vi "Q14070主界面Z100.vi"() -> ()   [LabVIEW 2013]
uses:
  <vilib>/Utility/error.llb/whitespace.ctl
  <vilib>/Utility/file.llb/Write To Spreadsheet File (string).vi
  <vilib>/Utility/file.llb/Write To Spreadsheet File (DBL).vi
  <vilib>/Utility/file.llb/Read From Spreadsheet File (DBL).vi
  <vilib>/Utility/file.llb/Read From Spreadsheet File (string).vi
panel:
  out "放行1":bool
  in  "流水号 3":dbl=22.0 min=1.0 format="%0#8_4g"
  out "打标内容 2":string
  out "PLC":bool
  out "本序已做":bool
  out "10rfid读取完成":bool
  out "10RFID读取触发":bool
  out "FGCS":string
  out "KSJJ":string
  out "10rfid":string
  out "上序不合格":bool
  out "上序合格":bool
  out "自动工步号Z110":dbl
  out "Z110工位操作状态":string
  out "芯片ID":string
  out "本序不合格":bool
  out "权限":string
  out "本序合格":bool
  in  "停止":bool
  in  "自动工步号":dbl
  out "产品选型":dbl
  out "Z100工位操作状态":string
  in  "联线按钮":bool
  in  "选项卡控件":enum32{"自动界面", "手动界面"}(tab)
  out "字符串":string
  in  "批次":string="A"
  in  "流水号 2":dbl=22.0 min=1.0 format="%0#8_4g"
  out "打标内容":string
  out "打标内容第二行":string
  in  "流水号":dbl min=1.0 format="%0#6_4g"
  out "打标内容第一行":string
  in  "放行":bool
  in  "阻挡":bool
  in  "Z110旋转气缸回原":bool
  in  "Z110旋转气缸旋转":bool
  in  "Z100上阻挡器":bool
  in  "Z100下阻挡器":bool
  in  "Z100顶升气缸上升":bool
  in  "Z100顶升气缸下降":bool
  in  "Z110下阻挡器":bool
  in  "Z110顶升气缸上升":bool
  in  "Z110顶升气缸下降":bool
  out "放行按钮":bool
  out "启动按钮":bool
  out "复位按钮":bool
  out "自动手动旋钮":bool
  out "急停按钮":bool
  out "本工位检测":bool
  out "Z110下工位检测":bool
  out "Z110放行按钮":bool
  out "顶升气缸上位":bool
  out "上工位检测":bool
  out "Z110本工位检测":bool
  out "顶升气缸下位":bool
  out "Z110复位按钮":bool
  out "Z110旋转原位":bool
  out "Z110急停按钮":bool
  out "下工位检测":bool
  out "Z110顶升下位":bool
  out "Z110顶升上位":bool
  out "Z110旋转位":bool
  in  "打标完成":bool
  out "员工ID":string
  out "员工姓名":string
  in  "型号选择":u16(ring)=1 items=["J709", "J706", "J728"]
  in  "参数加载":bool
  out "产品ID":string="4BSHL07134CCA"
  # "芜湖机械转向器装配线"
  # "激光打标"
  # "Q14070机械转向器装配线"
  # "湖北唯思凌科装备制造有限公司 设计开发 (C)2015"
  # "J728"
  # "J709"
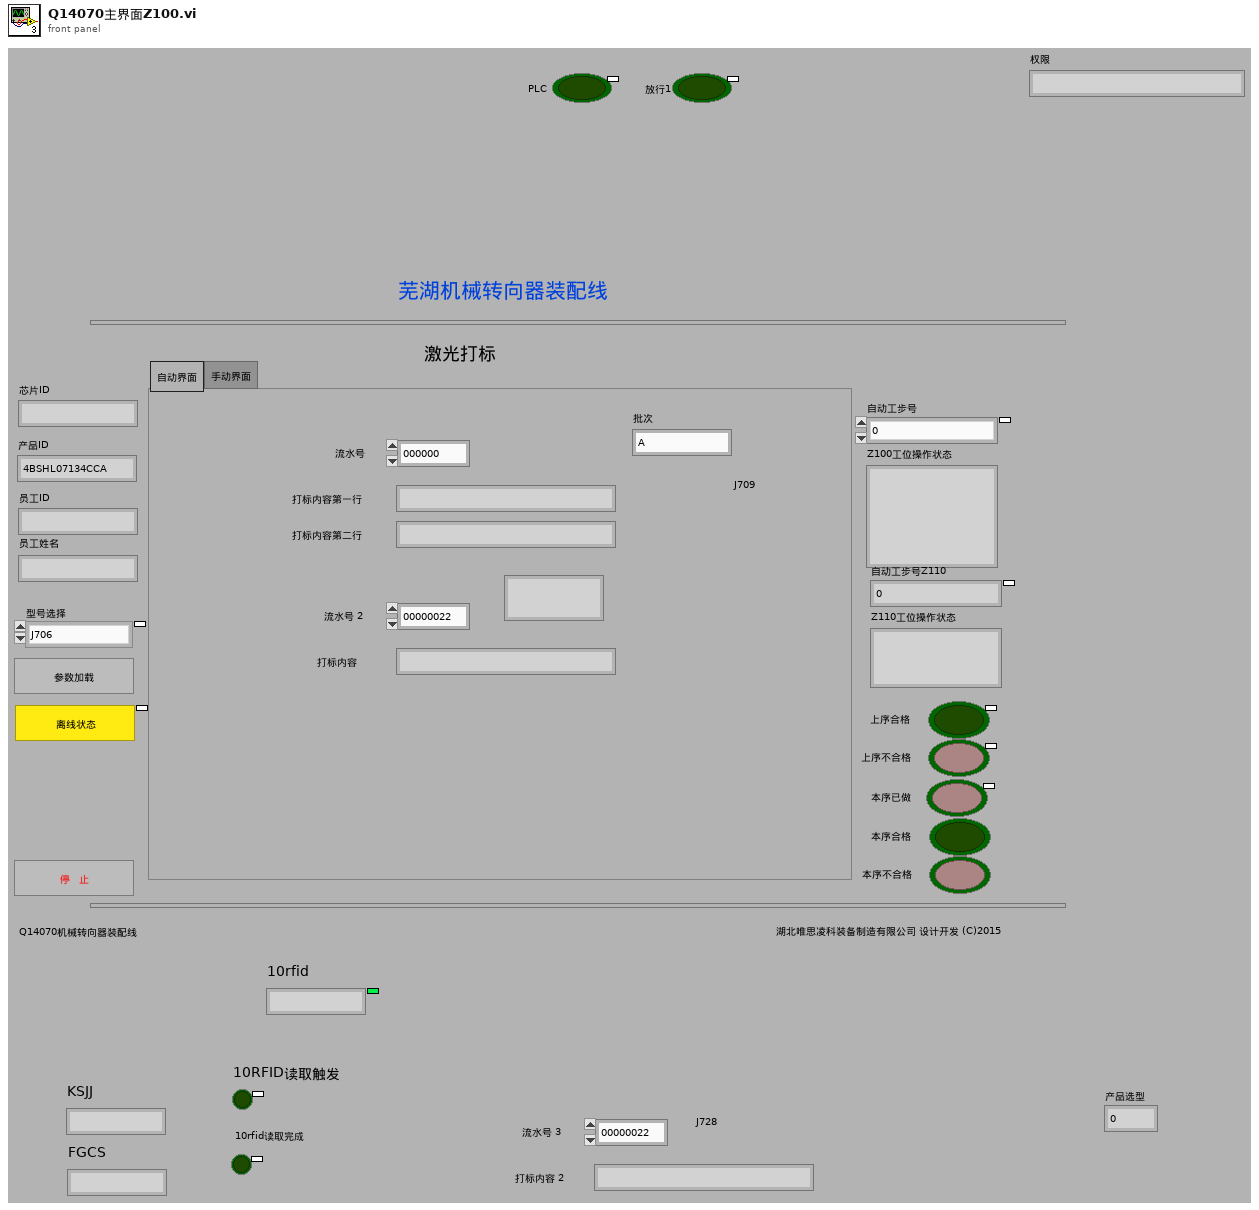
[diagram p1: front panel]
types:
  T1 = enum16{"open", "replace", "create", "open or create", "replace or create", "replace or create with confirmation"}
  T2 = typedef "whitespace.ctl" = u16
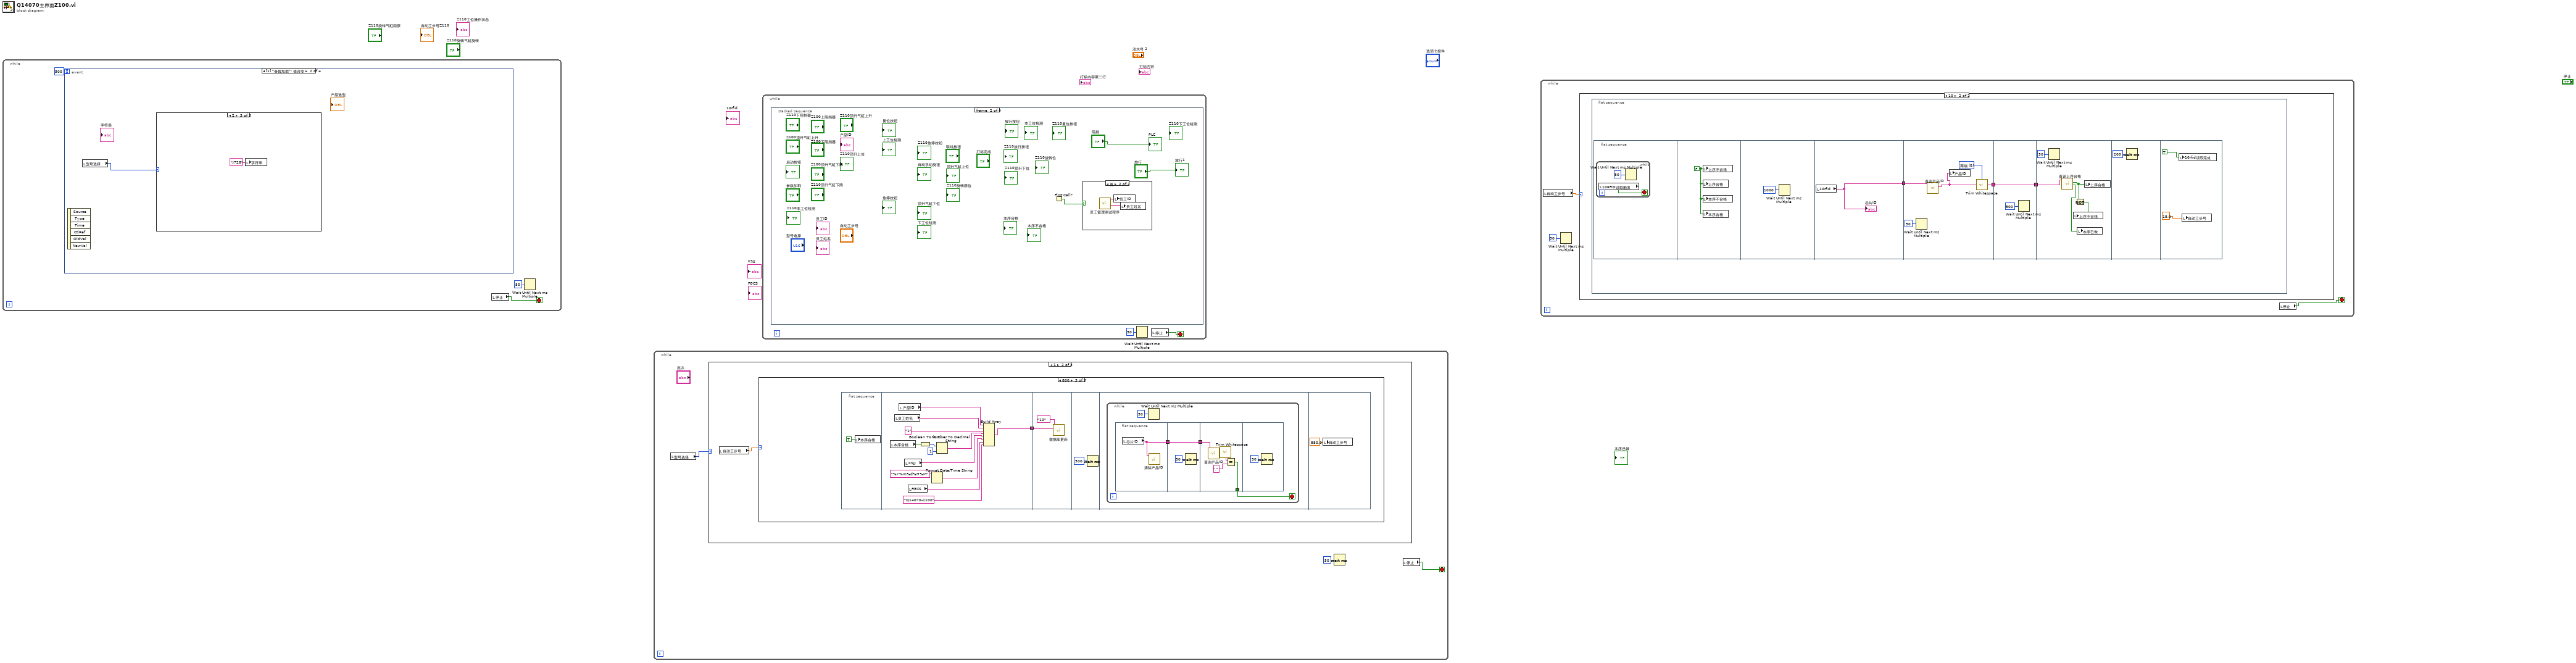
[diagram p0: block diagram]
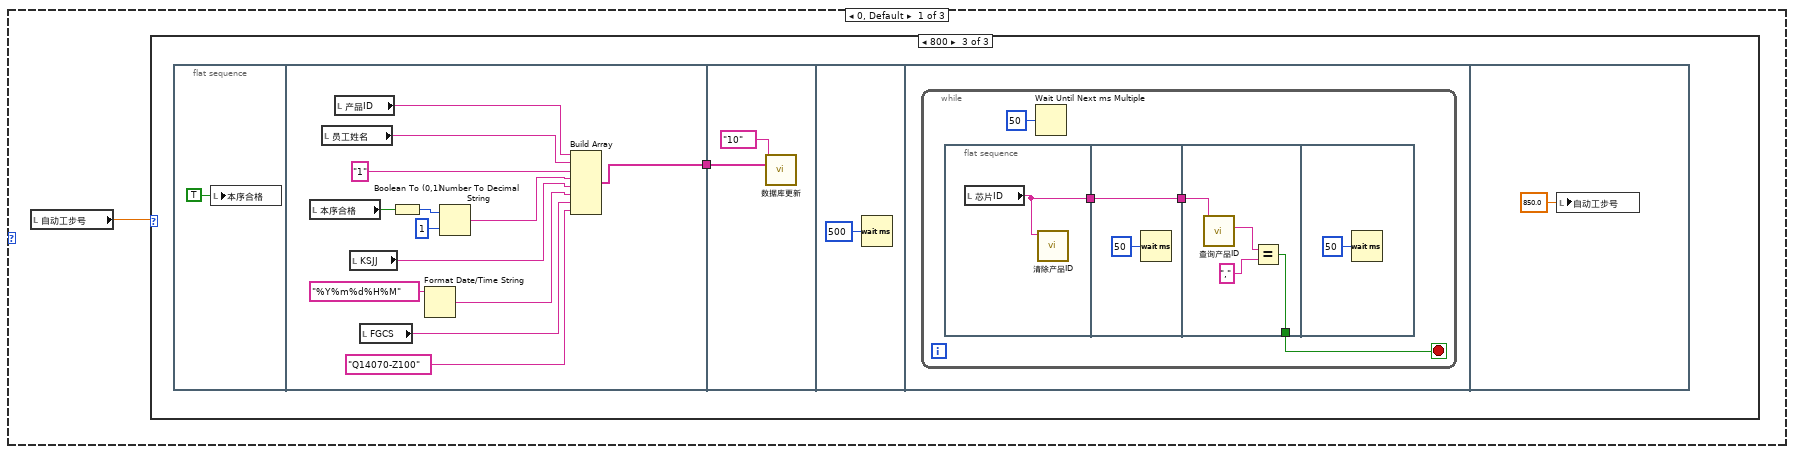
[diagram p2: hidden frame]
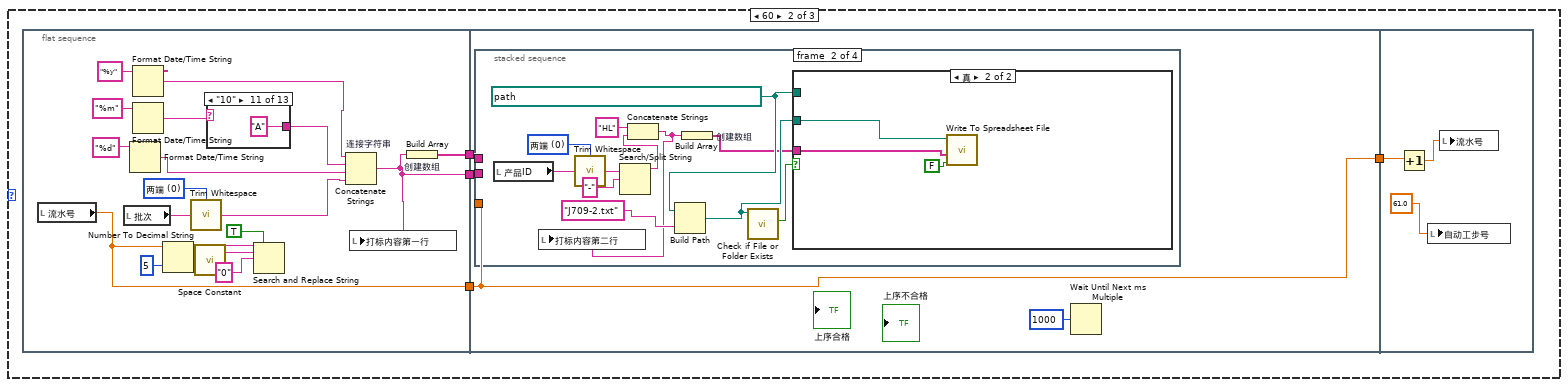
[diagram p4: hidden frame]
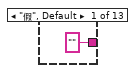
[diagram p5: hidden frame]
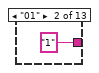
[diagram p6: hidden frame]
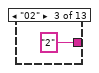
[diagram p7: hidden frame]
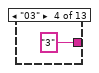
[diagram p8: hidden frame]
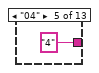
[diagram p9: hidden frame]
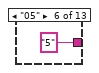
[diagram p10: hidden frame]
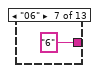
[diagram p11: hidden frame]
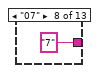
[diagram p12: hidden frame]
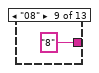
[diagram p13: hidden frame]
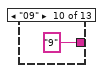
[diagram p14: hidden frame]
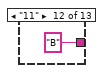
[diagram p15: hidden frame]
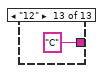
[diagram p16: hidden frame]
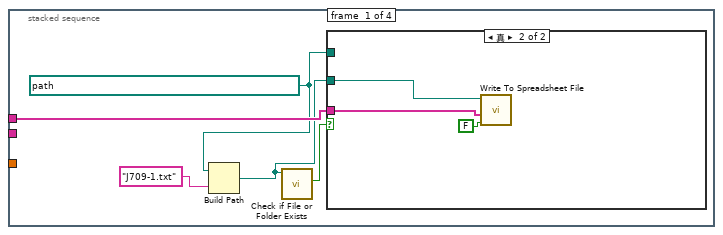
[diagram p17: hidden frame]
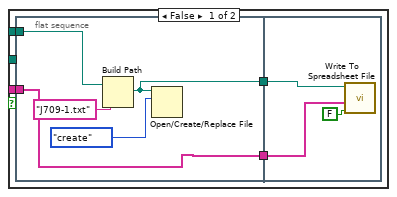
[diagram p18: hidden frame]
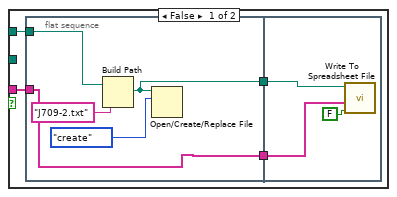
[diagram p19: hidden frame]
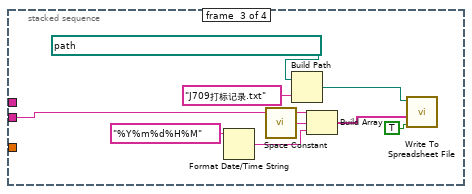
[diagram p20: hidden frame]
diagram:
  n1 = while {
    stop <- w1 stop-if-true
    n2 = event shown="[1] \"参数加载\": 值改变" {
      selector: _ -> [_ _ _ _]
      dyn-events: _ -> [_ _ _ _]
      timeout: 500 -> [_ _ _ _]
      event Timeout {
        n3 = event-data() -> ()  [unwired: 3 out]
      }
      event "参数加载": Value Change {
        n4 = event-data() -> ()  [unwired: 7 out]
        n5 = local read "型号选择"() -> (w4:u16)
        n6 = case shown="2" w4 {
          frame 0, Default {
          }
          frame 1 {
            n7 = local write "字符串"("J706" ("字符串")) -> ()
          }
          frame 2 {
            n8 = local write "字符串"("J728" ("字符串")) -> ()
          }
        }
      }
      event "停止": Value Change {
        n9 = event-data() -> ()  [unwired: 7 out]
        n10 = flat-sequence {
          frame #0 {
          }
          frame #1 {
            n11 = Wait Until Next ms Multiple(millisecond multiple=u32 1000 ("毫秒倍数")) -> ()  [unwired: 1 out]
          }
          frame #2 {
            n12 = Quit LabVIEW(quit? (T)=TRUE ("停止？(T)")) -> ()
          }
        }
      }
      event "产品ID": Value Change {
        n13 = event-data() -> ()  [unwired: 7 out]
        n14 = Format Date/Time String(time format string (%c)="%Y%m%d%H%M" ("时间格式字符串(%c)")) -> (date/time string=w9:string)  [unwired: 2 in]
        n15 = local write "KSJJ"(w9) -> ()
      }
    }
    n16 = local read "停止"() -> (w1:bool)
    n17 = Wait Until Next ms Multiple(millisecond multiple=u32 50 ("毫秒倍数")) -> ()  [unwired: 1 out]
  }
  n18 = while {
    stop <- w12 stop-if-true
    n19 = local read "型号选择"() -> (w13:u16)
    n20 = case shown="1" w13 {
      frame 0, Default {
        n21 = local read "自动工步号"() -> (w14:dbl)
        n22 = case shown="800" w14 {
          frame 0, Default {
          }
          frame 60 {
            n23 = flat-sequence {
              tunnel: [w31] -> w18
              tunnel: [w30] -> w17
              tunnel: [w20] -> w15
              tunnel: [w51] -> w16
              tunnel: w18 -> [w52]
              tunnel: w17 -> [w51]
              tunnel: w15 -> [w50]
              tunnel: w16 -> [w119]
              frame #0 {
                w25 = T2 0 items=["两端", "字符串首端", "字符串末端"] ("location (both)")
                n24 = local read "流水号"() -> (w30:dbl)
                n25 = local read "批次"() -> (w26:string)
                n26 = Format Date/Time String(time format string (%c)="%d" ("时间格式字符串(%c)")) -> (date/time string=w22:string)  [unwired: 2 in]
                n27 = Format Date/Time String(time format string (%c)="%y" ("时间格式字符串(%c)")) -> (date/time string=w19:string)  [unwired: 2 in]
                n28 = Format Date/Time String(time format string (%c)="%m" ("时间格式字符串(%c)")) -> (date/time string=w27:string)  [unwired: 2 in]
                n29 = Number To Decimal String(number=w30, width (-)=i16 5 ("宽度(-)")) -> (decimal integer string=w33:string)
                n30 = call <vilib>:"Trim Whitespace.vi"("string"=w26, "location (both)"=w25) -> ("trimmed string"=w21:string)
                n31 = call <vilib>:"Space Constant.vi"() -> ("String"=w35:string)
                n32 = case shown="\"10\"" w27 {
                  tunnel: ["" "1" "2" "3" "4" "5" "6" "7" "8" "9" "A" "B" "C"] -> w23
                  frame "假", Default {
                  }
                  frame "01" {
                  }
                  frame "02" {
                  }
                  frame "03" {
                  }
                  frame "04" {
                  }
                  frame "05" {
                  }
                  frame "06" {
                  }
                  frame "07" {
                  }
                  frame "08" {
                  }
                  frame "09" {
                  }
                  frame "10" {
                  }
                  frame "11" {
                  }
                  frame "12" {
                  }
                }
                n33 = Search and Replace String(replace all?=TRUE ("替换全部？(F)"), input string=w33, search string=w35, replace string="0" ("替换字符串(\"\")")) -> ()  [unwired: 4 in, 4 out]
                n34 = Concatenate Strings "连接字符串"(w19, w23, w22, w21) -> (w20:string)
                n35 = local write "打标内容第一行"(w20) -> ()
                n36 = Build Array "创建数组"(w20) -> (w31:string[])
              }
              frame #1 {
                n37 = stacked-sequence {
                  tunnel: w52 -> [w57 _ _ _]
                  tunnel: w51 -> [_ _ _ w112]
                  tunnel: w50 -> [_ _ w101 _]
                  frame #0 {
                    w55 = path "D:/Q14070-Z100人机界面/子VI/打标内容/J709" ("file path (dialog if empty)")
                    n38 = Build Path(base path=w55, name or relative path="J709-1.txt" ("名称或相对路径")) -> (appended path=w56:path)
                    n39 = call <vilib>:"Check if File or Folder Exists.vi"("path"=w56) -> ("file or folder exists?"=w58:bool)  [unwired: 8 in, 2 out]
                    n40 = case shown="真" w58 {
                      tunnel: w56 -> [_ w73]
                      tunnel: w55 -> [w62 _]
                      tunnel: w57 -> [w59 w71]
                      frame False {
                        n41 = flat-sequence {
                          tunnel: w62 -> [w67]
                          tunnel: [w64] -> w61
                          tunnel: [w63] -> w60
                          tunnel: w59 -> [w63]
                          tunnel: w61 -> [w69]
                          tunnel: w60 -> [w68]
                          frame #0 {
                            n42 = Build Path(base path=w67, name or relative path="J709-1.txt" ("名称或相对路径")) -> (appended path=w64:path)
                            n43 = Open/Create/Replace File ("打开/创建/替换文件")(file path (use dialog)=w64, operation (0:open)=T1."create" ("操作(0:open)")) -> ()  [unwired: 4 in, 3 out]
                          }
                          frame #1 {
                            n44 = call-poly <vilib>:"Write To Spreadsheet File.vi"("append to file? (new file:F)"=FALSE, "1D data"=w68, "file path (dialog if empty)"=w69) -> ()  [unwired: 5 in, 1 out]
                          }
                        }
                      }
                      frame True {
                        n45 = call-poly <vilib>:"Write To Spreadsheet File.vi"("append to file? (new file:F)"=FALSE, "1D data"=w71, "file path (dialog if empty)"=w73) -> ()  [unwired: 5 in, 1 out]
                      }
                    }
                  }
                  frame #1 {
                    w81 = T2 0 items=["两端", "字符串首端", "字符串末端"] ("location (both)")
                    w83 = path "D:/Q14070-Z100人机界面/子VI/打标内容/J709" ("file path (dialog if empty)")
                    n46 = local read "产品ID"() -> (w80:string)
                    n47 = call <vilib>:"Trim Whitespace.vi"("string"=w80, "location (both)"=w81) -> ("trimmed string"=w76:string)
                    n48 = Search/Split String(string=w76, search string/char (-)="-" ("搜索字符串/字符(-)")) -> (substring before match=w75:string)  [unwired: 1 in, 2 out]
                    n49 = Concatenate Strings ("连接字符串")("HL" ("字符串"), w75) -> (w77:string)
                    n50 = local write "打标内容第二行"(w77) -> ()
                    n51 = Build Path(base path=w83, name or relative path="J709-2.txt" ("名称或相对路径")) -> (appended path=w84:path)
                    n52 = Build Array "创建数组"(w77) -> (w78:string[])
                    n53 = call <vilib>:"Check if File or Folder Exists.vi"("path"=w84) -> ("file or folder exists?"=w85:bool)  [unwired: 8 in, 2 out]
                    n54 = case shown="真" w85 {
                      tunnel: w84 -> [_ w100]
                      tunnel: w83 -> [w89 _]
                      tunnel: w78 -> [w86 w98]
                      frame False {
                        n55 = flat-sequence {
                          tunnel: w89 -> [w94]
                          tunnel: [w92] -> w88
                          tunnel: [w91] -> w87
                          tunnel: w86 -> [w91]
                          tunnel: w88 -> [w96]
                          tunnel: w87 -> [w95]
                          frame #0 {
                            n56 = Build Path(base path=w94, name or relative path="J709-2.txt" ("名称或相对路径")) -> (appended path=w92:path)
                            n57 = Open/Create/Replace File ("打开/创建/替换文件")(file path (use dialog)=w92, operation (0:open)=T1."create" ("操作(0:open)")) -> ()  [unwired: 4 in, 3 out]
                          }
                          frame #1 {
                            n58 = call-poly <vilib>:"Write To Spreadsheet File.vi"("append to file? (new file:F)"=FALSE, "1D data"=w95, "file path (dialog if empty)"=w96) -> ()  [unwired: 5 in, 1 out]
                          }
                        }
                      }
                      frame True {
                        n59 = call-poly <vilib>:"Write To Spreadsheet File.vi"("append to file? (new file:F)"=FALSE, "1D data"=w98, "file path (dialog if empty)"=w100) -> ()  [unwired: 5 in, 1 out]
                      }
                    }
                  }
                  frame #2 {
                    n60 = Format Date/Time String(time format string (%c)="%Y%m%d%H%M" ("时间格式字符串(%c)")) -> (date/time string=w104:string)  [unwired: 2 in]
                    n61 = call <vilib>:"Space Constant.vi"() -> ("String"=w105:string)
                    n62 = Build Path(base path=path "D:/Q14070-Z100人机界面/子VI/打标内容/J709" ("file path (dialog if empty)"), name or relative path="J709打标记录.txt" ("名称或相对路径")) -> (appended path=w102:path)
                    n63 = Build Array(w101, w105, w104) -> (w103:string[])
                    n64 = call-poly <vilib>:"Write To Spreadsheet File.vi"("append to file? (new file:F)"=TRUE, "1D data"=w103, "file path (dialog if empty)"=w102) -> ()  [unwired: 5 in, 1 out]
                  }
                  frame #3 {
                    n65 = Increment(x=w112) -> (x+1=w111:dbl)
                    n66 = Build Array(w111) -> (w110:dbl[])
                    n67 = Build Path(base path=path "D:/Q14070-Z100人机界面/子VI/打标内容/J709" ("file path (dialog if empty)"), name or relative path="J709流水号.txt" ("名称或相对路径")) -> (appended path=w113:path)
                    n68 = call-poly <vilib>:"Write To Spreadsheet File.vi"("append to file? (new file:F)"=FALSE, "1D data"=w110, "file path (dialog if empty)"=w113) -> ()  [unwired: 5 in, 1 out]
                  }
                }
                n69 = Wait Until Next ms Multiple(millisecond multiple=u32 1000 ("毫秒倍数")) -> ()  [unwired: 1 out]
              }
              frame #2 {
                n70 = Increment(x=w119) -> (x+1=w118:dbl)
                n71 = local write "自动工步号"(61.0 ("打标工位工步号")) -> ()
                n72 = local write "流水号"(w118) -> ()
              }
            }
          }
          frame 800 {
            n73 = flat-sequence {
              tunnel: [w123] -> w120
              tunnel: w120 -> [w135]
              frame #0 {
                n74 = local write "本序合格"(TRUE ("本序合格")) -> ()
              }
              frame #1 {
                n75 = local read "本序合格"() -> (w122:bool)
                n76 = local read "员工姓名"() -> (w130:string)
                n77 = local read "产品ID"() -> (w131:string)
                n78 = local read "KSJJ"() -> (w127:string)
                n79 = local read "FGCS"() -> (w125:string)
                n80 = Boolean To (0,1)(Boolean=w122) -> (0, 1=w134:i16)
                n81 = Format Date/Time String(time format string (%c)="%Y%m%d%H%M" ("时间格式字符串(%c)")) -> (date/time string=w126:string)  [unwired: 2 in]
                n82 = Number To Decimal String(number=w134, width (-)=i16 1 ("宽度(-)")) -> (decimal integer string=w128:string)
                n83 = Build Array(w131, w130, "1", w128, w127, w126, w125, "Q14070-Z100") -> (w123:string[])
              }
              frame #2 {
                n84 = call "数据库更新.vi"("设备号"="10", "数据"=w135) -> ()  [unwired: 13 in, 1 out]
              }
              frame #3 {
                n85 = Wait (ms)(milliseconds to wait=u32 500 ("等待时间（毫秒）")) -> ()  [unwired: 1 out]
              }
              frame #4 {
                n86 = while {
                  stop <- w138 stop-if-true
                  n87 = flat-sequence {
                    tunnel: [w142] -> w139
                    tunnel: [w143] -> w140
                    tunnel: w139 -> [w143]
                    tunnel: w140 -> [w148]
                    tunnel: [w145] -> w138
                    frame #0 {
                      n88 = local read "芯片ID"() -> (w142:string)
                      n89 = call "清除产品ID.vi"("芯片编码"=w142) -> ()  [unwired: 10 in, 1 out]
                    }
                    frame #1 {
                      n90 = Wait (ms)(milliseconds to wait=u32 50 ("等待时间（毫秒）")) -> ()  [unwired: 1 out]
                    }
                    frame #2 {
                      n91 = call "查询产品ID.vi"("芯片编码"=w148) -> ("产品ID"=w146:string)  [unwired: 8 in, 2 out]
                      n92 = Equal?(x=w146, y=",") -> (x = y?=w145:bool)
                    }
                    frame #3 {
                      n93 = Wait (ms)(milliseconds to wait=u32 50 ("等待时间（毫秒）")) -> ()  [unwired: 1 out]
                    }
                  }
                  n94 = Wait Until Next ms Multiple(millisecond multiple=u32 50 ("毫秒倍数")) -> ()  [unwired: 1 out]
                }
              }
              frame #5 {
                n95 = local write "自动工步号"(850.0 ("自动工步号")) -> ()
              }
            }
          }
        }
      }
      frame 1 {
        n96 = local read "自动工步号"() -> (w151:dbl)
        n97 = case shown="800" w151 {
          frame 0, Default {
          }
          frame 60 {
            n98 = flat-sequence {
              tunnel: [w164] -> w156
              tunnel: [w163] -> w155
              tunnel: [w162] -> w154
              tunnel: [w171] -> w153
              tunnel: w156 -> [w173]
              tunnel: w155 -> [w171]
              tunnel: w154 -> [w172]
              tunnel: w153 -> [w212]
              tunnel: [w212] -> w152
              tunnel: w152 -> [w215]
              frame #0 {
                w160 = T2 0 items=["两端", "字符串首端", "字符串末端"] ("location (both)")
                n99 = local read "产品ID"() -> (w161:string)
                n100 = local read "流水号 2"() -> (w163:dbl)
                n101 = call <vilib>:"Trim Whitespace.vi"("string"=w161, "location (both)"=w160) -> ("trimmed string"=w159:string)
                n102 = Format Date/Time String(time format string (%c)="%y%m" ("时间格式字符串(%c)")) -> ()  [unwired: 2 in, 1 out]
                n103 = Number To Decimal String(number=w163, width (-)=i16 5 ("宽度(-)")) -> (decimal integer string=w166:string)
                n104 = call <vilib>:"Space Constant.vi"() -> ("String"=w168:string)
                n105 = Search/Split String(string=w159, search string/char (-)="-" ("搜索字符串/字符(-)")) -> (substring before match=w157:string)  [unwired: 1 in, 2 out]
                n106 = Search and Replace String(replace all?=TRUE ("替换全部？(F)"), input string=w166, search string=w168, replace string="0" ("替换字符串(\"\")")) -> ()  [unwired: 4 in, 4 out]
                n107 = Concatenate Strings "连接字符串"(w157) -> (w162:string)
                n108 = local write "打标内容"(w162) -> ()
                n109 = Build Array(w162) -> (w164:string[])
              }
              frame #1 {
                n110 = stacked-sequence {
                  tunnel: w173 -> [w178 _ _]
                  tunnel: w172 -> [_ w200 _]
                  tunnel: w171 -> [_ _ w207]
                  frame #0 {
                    w175 = path "D:/Q14070-Z100人机界面/子VI/打标内容/J706" ("file path (dialog if empty)")
                    n111 = Build Path(base path=w175, name or relative path="J706.txt" ("名称或相对路径")) -> (appended path=w177:path)
                    n112 = call <vilib>:"Check if File or Folder Exists.vi"("path"=w177) -> ("file or folder exists?"=w179:bool)  [unwired: 8 in, 2 out]
                    n113 = case shown="真" w179 {
                      tunnel: w177 -> [_ w194]
                      tunnel: w175 -> [w183 _]
                      tunnel: w178 -> [w180 w192]
                      frame False {
                        n114 = flat-sequence {
                          tunnel: w183 -> [w188]
                          tunnel: [w186] -> w182
                          tunnel: [w185] -> w181
                          tunnel: w180 -> [w185]
                          tunnel: w182 -> [w190]
                          tunnel: w181 -> [w189]
                          frame #0 {
                            n115 = Build Path(base path=w188, name or relative path="J706.txt" ("名称或相对路径")) -> (appended path=w186:path)
                            n116 = Open/Create/Replace File(file path (use dialog)=w186, operation (0:open)=T1."create" ("操作(0:open)")) -> ()  [unwired: 4 in, 3 out]
                          }
                          frame #1 {
                            n117 = call-poly <vilib>:"Write To Spreadsheet File.vi"("append to file? (new file:F)"=FALSE, "1D data"=w189, "file path (dialog if empty)"=w190) -> ()  [unwired: 5 in, 1 out]
                          }
                        }
                      }
                      frame True {
                        n118 = call-poly <vilib>:"Write To Spreadsheet File.vi"("append to file? (new file:F)"=FALSE, "1D data"=w192, "file path (dialog if empty)"=w194) -> ()  [unwired: 5 in, 1 out]
                      }
                    }
                  }
                  frame #1 {
                    n119 = Format Date/Time String(time format string (%c)="%Y%m%d%H%M" ("时间格式字符串(%c)")) -> (date/time string=w198:string)  [unwired: 2 in]
                    n120 = call <vilib>:"Space Constant.vi"() -> ("String"=w199:string)
                    n121 = Build Path(base path=path "D:/Q14070-Z100人机界面/子VI/打标内容/J706" ("file path (dialog if empty)"), name or relative path="J706打标记录.txt" ("名称或相对路径")) -> (appended path=w196:path)
                    n122 = Build Array(w200, w199, w198) -> (w197:string[])
                    n123 = call-poly <vilib>:"Write To Spreadsheet File.vi"("append to file? (new file:F)"=TRUE, "1D data"=w197, "file path (dialog if empty)"=w196) -> ()  [unwired: 5 in, 1 out]
                  }
                  frame #2 {
                    n124 = Increment(x=w207) -> (x+1=w206:dbl)
                    n125 = Build Array(w206) -> (w205:dbl[])
                    n126 = Build Path(base path=path "D:/Q14070-Z100人机界面/子VI/打标内容/J706" ("file path (dialog if empty)"), name or relative path="J706流水号.txt" ("名称或相对路径")) -> (appended path=w208:path)
                    n127 = call-poly <vilib>:"Write To Spreadsheet File.vi"("append to file? (new file:F)"=FALSE, "1D data"=w205, "file path (dialog if empty)"=w208) -> ()  [unwired: 5 in, 1 out]
                  }
                }
                n128 = Wait Until Next ms Multiple(millisecond multiple=u32 1000 ("毫秒倍数")) -> ()  [unwired: 1 out]
              }
              frame #2 {
                n129 = Wait (ms)(milliseconds to wait=u32 1000 ("等待时间（毫秒）")) -> ()  [unwired: 1 out]
              }
              frame #3 {
                n130 = Increment(x=w215) -> (x+1=w214:dbl)
                n131 = local write "自动工步号"(61.0 ("打标工位工步号")) -> ()
                n132 = local write "流水号 2"(w214) -> ()
              }
            }
          }
          frame 800 {
            n133 = flat-sequence {
              tunnel: [w219] -> w216
              tunnel: w216 -> [w231]
              frame #0 {
                n134 = local write "本序合格"(TRUE ("本序合格")) -> ()
              }
              frame #1 {
                n135 = local read "本序合格"() -> (w218:bool)
                n136 = local read "员工姓名"() -> (w226:string)
                n137 = local read "产品ID"() -> (w227:string)
                n138 = local read "KSJJ"() -> (w223:string)
                n139 = local read "FGCS"() -> (w221:string)
                n140 = Boolean To (0,1)(Boolean=w218) -> (0, 1=w230:i16)
                n141 = Format Date/Time String(time format string (%c)="%Y%m%d%H%M" ("时间格式字符串(%c)")) -> (date/time string=w222:string)  [unwired: 2 in]
                n142 = Number To Decimal String(number=w230, width (-)=i16 1 ("宽度(-)")) -> (decimal integer string=w224:string)
                n143 = Build Array(w227, w226, "1", w224, w223, w222, w221, "Q14070-Z100") -> (w219:string[])
              }
              frame #2 {
                n144 = call "数据库更新.vi"("设备号"="10", "数据"=w231) -> ()  [unwired: 13 in, 1 out]
              }
              frame #3 {
                n145 = Wait (ms)(milliseconds to wait=u32 500 ("等待时间（毫秒）")) -> ()  [unwired: 1 out]
              }
              frame #4 {
                n146 = while {
                  stop <- w234 stop-if-true
                  n147 = flat-sequence {
                    tunnel: [w238] -> w235
                    tunnel: [w239] -> w236
                    tunnel: w235 -> [w239]
                    tunnel: w236 -> [w245]
                    tunnel: [w242] -> w234
                    frame #0 {
                      n148 = local read "芯片ID"() -> (w238:string)
                      n149 = call "清除产品ID.vi"("芯片编码"=w238) -> ()  [unwired: 10 in, 1 out]
                    }
                    frame #1 {
                      n150 = Wait (ms)(milliseconds to wait=u32 50 ("等待时间（毫秒）")) -> ()  [unwired: 1 out]
                    }
                    frame #2 {
                      n151 = call "查询产品ID.vi"("芯片编码"=w245) -> ("产品ID"=w243:string)  [unwired: 8 in, 2 out]
                      n152 = call <vilib>:"Trim Whitespace.vi"("string"=w243) -> ("trimmed string"=w241:string)  [unwired: 1 in]
                      n153 = Equal?(x=w241, y=",") -> (x = y?=w242:bool)
                    }
                    frame #3 {
                      n154 = Wait (ms)(milliseconds to wait=u32 50 ("等待时间（毫秒）")) -> ()  [unwired: 1 out]
                    }
                  }
                  n155 = Wait Until Next ms Multiple(millisecond multiple=u32 50 ("毫秒倍数")) -> ()  [unwired: 1 out]
                }
              }
              frame #5 {
                n156 = local write "自动工步号"(850.0 ("自动工步号")) -> ()
              }
            }
          }
        }
      }
      frame 2 {
        n157 = local read "自动工步号"() -> (w248:dbl)
        n158 = case shown="60" w248 {
          frame 0, Default {
          }
          frame 60 {
            n159 = flat-sequence {
              tunnel: [w260] -> w252
              tunnel: [w253] -> w251
              tunnel: [w259] -> w250
              tunnel: [w267] -> w249
              tunnel: w252 -> [w269]
              tunnel: w251 -> [w267]
              tunnel: w250 -> [w268]
              tunnel: w249 -> [w309]
              frame #0 {
                w257 = T2 0 items=["两端", "字符串首端", "字符串末端"] ("location (both)")
                n160 = local read "产品ID"() -> (w258:string)
                n161 = local read "流水号 2"() -> (w253:dbl)
                n162 = call <vilib>:"Trim Whitespace.vi"("string"=w258, "location (both)"=w257) -> ("trimmed string"=w256:string)
                n163 = Format Date/Time String(time format string (%c)="%y%m" ("时间格式字符串(%c)")) -> ()  [unwired: 2 in, 1 out]
                n164 = Number To Decimal String(number=w253, width (-)=i16 5 ("宽度(-)")) -> (decimal integer string=w262:string)
                n165 = call <vilib>:"Space Constant.vi"() -> ("String"=w264:string)
                n166 = Search/Split String(string=w256, search string/char (-)="-" ("搜索字符串/字符(-)")) -> (substring before match=w254:string)  [unwired: 1 in, 2 out]
                n167 = Search and Replace String(replace all?=TRUE ("替换全部？(F)"), input string=w262, search string=w264, replace string="0" ("替换字符串(\"\")")) -> ()  [unwired: 4 in, 4 out]
                n168 = Concatenate Strings "连接字符串"(w254) -> (w259:string)
                n169 = local write "打标内容"(w259) -> ()
                n170 = Build Array(w259) -> (w260:string[])
              }
              frame #1 {
                n171 = stacked-sequence {
                  tunnel: w269 -> [w274 _ _]
                  tunnel: w268 -> [_ w296 _]
                  tunnel: w267 -> [_ _ w303]
                  frame #0 {
                    w271 = path "D:/Q14070-Z100人机界面/子VI/打标内容/J728" ("file path (dialog if empty)")
                    n172 = Build Path(base path=w271, name or relative path="J728.txt" ("名称或相对路径")) -> (appended path=w273:path)
                    n173 = call <vilib>:"Check if File or Folder Exists.vi"("path"=w273) -> ("file or folder exists?"=w275:bool)  [unwired: 8 in, 2 out]
                    n174 = case shown="假" w275 {
                      tunnel: w273 -> [_ w290]
                      tunnel: w271 -> [w279 _]
                      tunnel: w274 -> [w276 w288]
                      frame False {
                        n175 = flat-sequence {
                          tunnel: w279 -> [w284]
                          tunnel: [w282] -> w278
                          tunnel: [w281] -> w277
                          tunnel: w276 -> [w281]
                          tunnel: w278 -> [w286]
                          tunnel: w277 -> [w285]
                          frame #0 {
                            n176 = Build Path(base path=w284, name or relative path="J728.txt" ("名称或相对路径")) -> (appended path=w282:path)
                            n177 = Open/Create/Replace File(file path (use dialog)=w282, operation (0:open)=T1."create" ("操作(0:open)")) -> ()  [unwired: 4 in, 3 out]
                          }
                          frame #1 {
                            n178 = call-poly <vilib>:"Write To Spreadsheet File.vi"("append to file? (new file:F)"=FALSE, "1D data"=w285, "file path (dialog if empty)"=w286) -> ()  [unwired: 5 in, 1 out]
                          }
                        }
                      }
                      frame True {
                        n179 = call-poly <vilib>:"Write To Spreadsheet File.vi"("append to file? (new file:F)"=FALSE, "1D data"=w288, "file path (dialog if empty)"=w290) -> ()  [unwired: 5 in, 1 out]
                      }
                    }
                  }
                  frame #1 {
                    n180 = Format Date/Time String(time format string (%c)="%Y%m%d%H%M" ("时间格式字符串(%c)")) -> (date/time string=w294:string)  [unwired: 2 in]
                    n181 = call <vilib>:"Space Constant.vi"() -> ("String"=w295:string)
                    n182 = Build Path(base path=path "D:/Q14070-Z100人机界面/子VI/打标内容/J728" ("file path (dialog if empty)"), name or relative path="J728打标记录.txt" ("名称或相对路径")) -> (appended path=w292:path)
                    n183 = Build Array(w296, w295, w294) -> (w293:string[])
                    n184 = call-poly <vilib>:"Write To Spreadsheet File.vi"("append to file? (new file:F)"=TRUE, "1D data"=w293, "file path (dialog if empty)"=w292) -> ()  [unwired: 5 in, 1 out]
                  }
                  frame #2 {
                    n185 = Increment(x=w303) -> (x+1=w302:dbl)
                    n186 = Build Array(w302) -> (w301:dbl[])
                    n187 = Build Path(base path=path "D:/Q14070-Z100人机界面/子VI/打标内容/J728" ("file path (dialog if empty)"), name or relative path="J728流水号.txt" ("名称或相对路径")) -> (appended path=w304:path)
                    n188 = call-poly <vilib>:"Write To Spreadsheet File.vi"("append to file? (new file:F)"=FALSE, "1D data"=w301, "file path (dialog if empty)"=w304) -> ()  [unwired: 5 in, 1 out]
                  }
                }
                n189 = Wait Until Next ms Multiple(millisecond multiple=u32 1000 ("毫秒倍数")) -> ()  [unwired: 1 out]
              }
              frame #2 {
                n190 = Increment(x=w309) -> (x+1=w308:dbl)
                n191 = local write "自动工步号"(61.0 ("打标工位工步号")) -> ()
                n192 = local write "流水号 3"(w308) -> ()
              }
            }
          }
          frame 800 {
            n193 = flat-sequence {
              tunnel: [w313] -> w310
              tunnel: w310 -> [w325]
              frame #0 {
                n194 = local write "本序合格"(TRUE ("本序合格")) -> ()
              }
              frame #1 {
                n195 = local read "本序合格"() -> (w312:bool)
                n196 = local read "员工姓名"() -> (w320:string)
                n197 = local read "产品ID"() -> (w321:string)
                n198 = local read "KSJJ"() -> (w317:string)
                n199 = local read "FGCS"() -> (w315:string)
                n200 = Boolean To (0,1)(Boolean=w312) -> (0, 1=w324:i16)
                n201 = Format Date/Time String(time format string (%c)="%Y%m%d%H%M" ("时间格式字符串(%c)")) -> (date/time string=w316:string)  [unwired: 2 in]
                n202 = Number To Decimal String(number=w324, width (-)=i16 1 ("宽度(-)")) -> (decimal integer string=w318:string)
                n203 = Build Array(w321, w320, "1", w318, w317, w316, w315, "Q14070-Z100") -> (w313:string[])
              }
              frame #2 {
                n204 = call "数据库更新.vi"("设备号"="10", "数据"=w325) -> ()  [unwired: 13 in, 1 out]
              }
              frame #3 {
                n205 = Wait (ms)(milliseconds to wait=u32 500 ("等待时间（毫秒）")) -> ()  [unwired: 1 out]
              }
              frame #4 {
                n206 = while {
                  stop <- w328 stop-if-true
                  n207 = flat-sequence {
                    tunnel: [w332] -> w329
                    tunnel: [w333] -> w330
                    tunnel: w329 -> [w333]
                    tunnel: w330 -> [w338]
                    tunnel: [w335] -> w328
                    frame #0 {
                      n208 = local read "芯片ID"() -> (w332:string)
                      n209 = call "清除产品ID.vi"("芯片编码"=w332) -> ()  [unwired: 10 in, 1 out]
                    }
                    frame #1 {
                      n210 = Wait (ms)(milliseconds to wait=u32 50 ("等待时间（毫秒）")) -> ()  [unwired: 1 out]
                    }
                    frame #2 {
                      n211 = call "查询产品ID.vi"("芯片编码"=w338) -> ("产品ID"=w336:string)  [unwired: 8 in, 2 out]
                      n212 = Equal?(x=w336, y=",") -> (x = y?=w335:bool)
                    }
                    frame #3 {
                      n213 = Wait (ms)(milliseconds to wait=u32 50 ("等待时间（毫秒）")) -> ()  [unwired: 1 out]
                    }
                  }
                  n214 = Wait Until Next ms Multiple(millisecond multiple=u32 50 ("毫秒倍数")) -> ()  [unwired: 1 out]
                }
              }
              frame #5 {
                n215 = local write "自动工步号"(850.0 ("自动工步号")) -> ()
              }
            }
          }
        }
      }
    }
    n216 = Wait (ms)(milliseconds to wait=u32 50 ("等待时间（毫秒）")) -> ()  [unwired: 1 out]
    n217 = local read "停止"() -> (w12:bool)
  }
  n218 = while {
    stop <- w341 stop-if-true
    n219 = stacked-sequence {
      frame #0 {
        n220 = disable-structure shown="禁用" {
          frame Disabled {
            n221 = First Call?() -> (First Call?: T/F=w343:bool)
            n222 = case shown="真" w343 {
              frame False {
              }
              frame True {
                n223 = call-poly <vilib>:"Read From Spreadsheet File.vi"("file path (dialog if empty)"=path "\\\\Q113600\\参数/00/管理策略.txt" ("基路径")) -> ("all rows"=w346:string[][])  [unwired: 3 in, 7 out]
                n224 = Index Array(array=w346, index (col)=1 ("索引 (行)")) -> (element=w347:string[])  [unwired: 1 in]
                n225 = Index Array(array=w347, index=0 ("索引")) -> (element=w349:string)
                n226 = Equal?(x=w349, y="1") -> (x = y?=w351:bool)
                n227 = case shown="真" w351 {
                  frame False {
                  }
                  frame True {
                    n228 = while {
                      stop <- w353 continue-if-true
                      n229 = flat-sequence {
                        tunnel: [w359] -> w354
                        tunnel: w354 -> [w363]
                        tunnel: [w363] -> w353
                        frame #0 {
                          w357 = T2 0 items=["两端", "字符串首端", "字符串末端"] ("location (both)")
                          n230 = local read "权限"() -> (w355:string)
                          n231 = call <vilib>:"Trim Whitespace.vi"("string"=w355, "location (both)"=w357) -> ("trimmed string"=w356:string)
                          n232 = Not Equal?(x=w356, y="0") -> (x != y?=w358:bool)
                          n233 = Not Equal?(x=w356, y="3") -> (x != y?=w362:bool)
                          n234 = And(x=w358, y=w362) -> (x .and. y?=w359:bool)
                        }
                        frame #1 {
                          n235 = call "请输入员工ID"("Enable"=w363) -> ("请输入员工ID"=w364:string, "确定"=w365:bool)  [unwired: 1 in, 16 out]
                          n236 = Wait (ms)(milliseconds to wait=u32 200 ("等待时间（毫秒）")) -> ()  [unwired: 1 out]
                          n237 = case shown="真" w365 {
                            tunnel: w364 -> [_ w367]
                            frame False {
                            }
                            frame True {
                              n238 = local write "员工ID"(w367) -> ()
                              n239 = call "查询员工.vi"("员工ID"=w367) -> ("权限"=w370:string, "姓名"=w371:string)  [unwired: 7 in, 2 out]
                              n240 = call <vilib>:"Trim Whitespace.vi"("string"=w370) -> ("trimmed string"=w369:string)  [unwired: 1 in]
                              n241 = call <vilib>:"Trim Whitespace.vi"("string"=w371) -> ("trimmed string"=w368:string)  [unwired: 1 in]
                              n242 = local write "员工姓名"(w368) -> ()
                              n243 = local write "权限"(w369) -> ()
                            }
                          }
                        }
                      }
                      n244 = Wait (ms)(milliseconds to wait=u32 200 ("等待时间（毫秒）")) -> ()  [unwired: 1 out]
                    }
                  }
                }
              }
            }
          }
          frame Enabled {
          }
        }
      }
      frame #1 {
        n245 = First Call?() -> (First Call?: T/F=w374:bool)
        n246 = case shown="真" w374 {
          frame False {
          }
          frame True {
            n247 = call "员工管理测试程序.vi"() -> ("员工姓名"=w376:string, "员工ID"=w375:string)  [unwired: 10 in]
            n248 = local write "员工ID"(w375) -> ()
            n249 = local write "员工姓名"(w376) -> ()
          }
        }
        "PLC" <- "阻挡"
        "放行1" <- "放行"
      }
      frame #2 {
        n250 = local read "自动工步号"() -> (w378:dbl)
        n251 = case shown="0, 默认" w378 {
          tunnel: [w379 "" ("Z100工位操作状态")] -> w377
          frame 0, Default {
            n252 = local read "联线按钮"() -> (w380:bool)
            n253 = case shown="假" w380 {
              tunnel: ["等待工件" ("Z100工位操作状态") "等待扫描条码" ("Z100工位操作状态")] -> w379
              frame False {
              }
              frame True {
              }
            }
          }
          frame 10 {
          }
        }
        "Z100工位操作状态" <- w377
      }
      frame #3 {
        n254 = First Call?() -> (First Call?: T/F=w384:bool)
        n255 = case shown="真" w384 {
          frame False {
          }
          frame True {
            n256 = Build Path(base path=path "D:/Q14070-Z100人机界面/子VI/打标内容/J709" ("file path (dialog if empty)"), name or relative path="J709流水号.txt" ("名称或相对路径")) -> (appended path=w394:path)
            n257 = Build Path ("创建路径")(base path=path "D:/Q14070-Z100人机界面/子VI/打标内容/J706" ("file path (dialog if empty)"), name or relative path="J706流水号.txt" ("名称或相对路径")) -> (appended path=w388:path)
            n258 = call-poly <vilib>:"Read From Spreadsheet File.vi"("file path (dialog if empty)"=w394) -> ("first row"=w393:dbl[])  [unwired: 6 in, 4 out]
            n259 = call-poly <vilib>:"Read From Spreadsheet File.vi"("file path (dialog if empty)"=w388) -> ("first row"=w389:dbl[])  [unwired: 6 in, 4 out]
            n260 = Index Array(array=w393, index=0 ("索引")) -> (element=w391:dbl)
            n261 = Index Array(array=w389, index=0 ("索引")) -> (element=w385:dbl)
            n262 = local write "流水号"(w391) -> ()
            n263 = local write "流水号 2"(w385) -> ()
          }
        }
      }
    }
    n264 = Wait Until Next ms Multiple(millisecond multiple=u32 50 ("毫秒倍数")) -> ()  [unwired: 1 out]
    n265 = local read "停止"() -> (w341:bool)
  }
  n266 = while {
    stop <- w398 stop-if-true
    n267 = local read "自动工步号"() -> (w397:dbl)
    n268 = Wait Until Next ms Multiple(millisecond multiple=u32 50 ("毫秒倍数")) -> ()  [unwired: 1 out]
    n269 = case shown="10" w397 {
      frame 0, Default {
      }
      frame 10 {
        n270 = flat-sequence {
          frame #0 {
            n271 = flat-sequence {
              tunnel: [w407] -> w402
              tunnel: [w410] -> w401
              tunnel: w402 -> [w409]
              tunnel: w401 -> [w414]
              tunnel: [w414] -> w400
              tunnel: w400 -> [w418]
              frame #0 {
                n272 = while {
                  stop <- w403 stop-if-true
                  n273 = local read "10RFID读取触发"() -> (w403:bool)
                  n274 = Wait Until Next ms Multiple(millisecond multiple=u32 50 ("毫秒倍数")) -> ()  [unwired: 1 out]
                }
              }
              frame #1 {
                w405 = FALSE ("上序不合格")
                n275 = local write "上序不合格"(w405) -> ()
                n276 = local write "上序合格"(w405) -> ()
                n277 = local write "本序不合格"(w405) -> ()
                n278 = local write "本序合格"(w405) -> ()
              }
              frame #2 {
                n279 = Wait Until Next ms Multiple(millisecond multiple=u32 1000 ("毫秒倍数")) -> ()  [unwired: 1 out]
              }
              frame #3 {
                n280 = local read "10rfid"() -> (w407:string)
                "芯片ID" <- w407
              }
              frame #4 {
                w411 = T2 0 items=["两端", "字符串首端", "字符串末端"] ("location (both)")
                n281 = Wait Until Next ms Multiple(millisecond multiple=u32 50 ("毫秒倍数")) -> ()  [unwired: 1 out]
                n282 = call "查询产品ID.vi"("芯片编码"=w409) -> ("产品ID"=w408:string)  [unwired: 8 in, 2 out]
                n283 = local write "产品ID"(w408) -> ()
                n284 = call <vilib>:"Trim Whitespace.vi"("string"=w408, "location (both)"=w411) -> ("trimmed string"=w410:string)
              }
              frame #5 {
                n285 = Wait Until Next ms Multiple(millisecond multiple=u32 500 ("毫秒倍数")) -> ()  [unwired: 1 out]
              }
              frame #6 {
                n286 = Wait Until Next ms Multiple(millisecond multiple=u32 50 ("毫秒倍数")) -> ()  [unwired: 1 out]
                n287 = call "查询上序合格.vi"("产品ID"=w418) -> ("本序已做"=w415:bool, "上序合格"=w417:bool)  [unwired: 8 in, 1 out]
                n288 = Not(x=w417) -> (.not. x?=w416:bool)
                n289 = local write "上序不合格"(w416) -> ()
                n290 = local write "本序已做"(w415) -> ()
                n291 = local write "上序合格"(w417) -> ()
              }
              frame #7 {
                n292 = Wait (ms)(milliseconds to wait=u32 200 ("等待时间（毫秒）")) -> ()  [unwired: 1 out]
              }
              frame #8 {
                n293 = local write "10rfid读取完成"(TRUE ("RFID读取完成")) -> ()
                n294 = local write "自动工步号"(15.0 ("工步号")) -> ()
              }
            }
          }
        }
      }
    }
    n295 = local read "停止"() -> (w398:bool)
  }
